vi "Get Key.vi"(10 "key":string, 11 "section data":T1) -> (0 "key exists?":bool=TRUE, 1 "comment":string, 2 "value":string, 3 "section data out":T1, 4 "key index":i32)   [LabVIEW 2020, in "NI_LVConfig.lvlib"]
uses:
  <vilib>/Utility/config.llb/NI_LVConfig.lvlib
  <vilib>/Utility/config.llb/Section.ctl
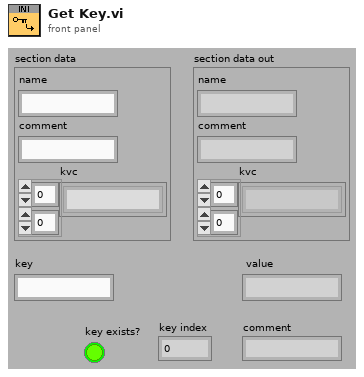
[diagram p1: front panel]
types:
  T1 = typedef "NI_LVConfig.lvlib/Section.ctl" = cluster{"name":string, "comment":string, "kvc":string[][]}
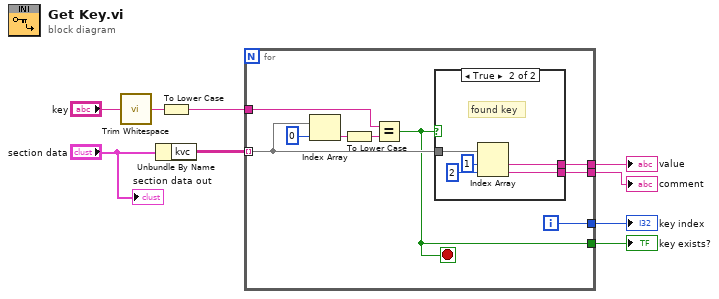
[diagram p0: block diagram]
diagram:
  n1 = call <vilib>:"Trim Whitespace.vi"("string"="key") -> ("trimmed string"=w2:string)  [unwired: 1 in]
  n2 = Unbundle By Name("section data") -> ("kvc"=w4:string[][])
  n3 = To Lower Case(string=w2) -> (all lower case string=w1:string)
  n4 = for {
    tunnel: w4 -> [w12] mode=indexing
    tunnel: w1 -> [w17]
    tunnel: [w10] -> w9
    tunnel: [w16] -> w8
    tunnel: [w11] -> w7
    tunnel: [w15] -> w5
    i -> [w11]
    stop <- w10 stop-if-true
    n5 = Index Array(array=w12, index=0) -> (element=w13:string)
    n6 = To Lower Case(string=w13) -> (all lower case string=w14:string)
    n7 = Equal?(x=w17, y=w14) -> (x = y?=w10:bool)
    n8 = case shown="True" w10 {
      tunnel: w12 -> [_ w22]
      tunnel: [_ w21] -> w16
      tunnel: [_ w19] -> w15
      frame False {
      }
      frame True {
        # "found key"
        n9 = Index Array(array=w22, index #1=1 ("index"), index #2=2 ("index")) -> (element #1=w21:string, element #2=w19:string)
      }
    }
  }
  "key exists?" <- w9
  "value" <- w8
  "key index" <- w7
  "comment" <- w5
  "section data out" <- "section data"
